vi "csmdoc_load vi description map.vi"(8 "Error in":errorcluster caption="Error in (no error)", 11 "Path":path=path "D:/github/JKI-State-Machine-Plus/.doc/VI Description.md") -> (0 "Error out":errorcluster, 1 "text":string, 2 "variant 2":variant, 3 "variant":variant)   [LabVIEW 2017, in "csmdoc.lvlib"]
uses:
  csmdoc.lvlib
  Communicable State Machine.lvlib
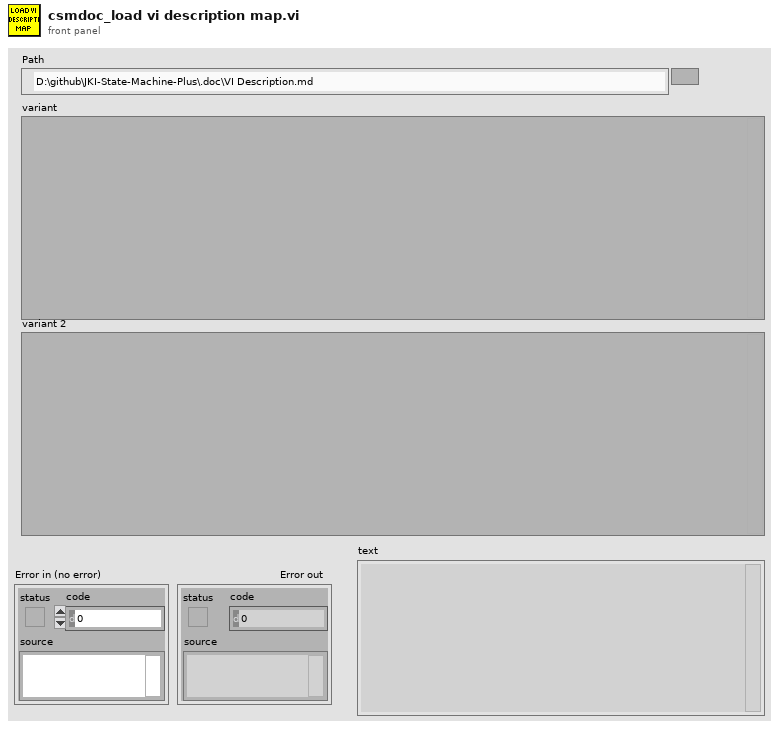
[diagram p1: front panel]
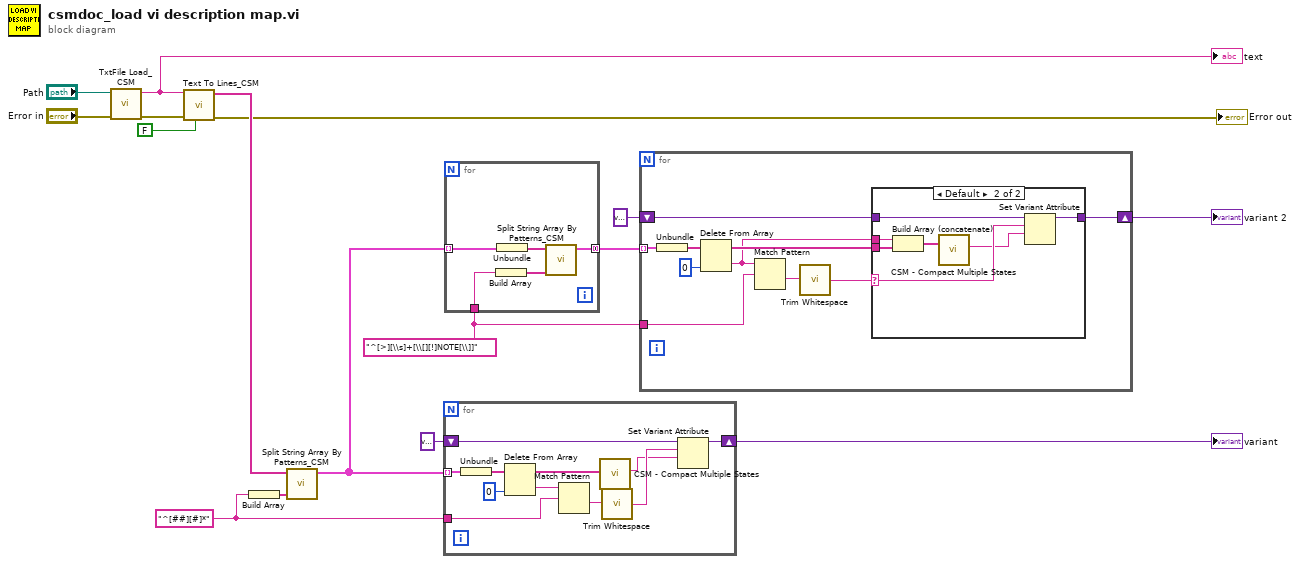
[diagram p0: block diagram]
diagram:
  w2 = "^[>][\\s]+[\\[][!]NOTE[\\]]" ("delimited string")
  w12 = "^[##][#]*" ("delimited string")
  n1 = call "TxtFile Load_CSM.vi"("error in (no error)"="Error in", "Path"="Path") -> ("error out"=w15:errorcluster, "text"=w14:string)  [unwired: 8 in]
  "text" <- w14
  n2 = call "Text To Lines_CSM.vi"("Remove Empty Lines?(T)"=FALSE, "error in (no error)"=w15, "string"=w14) -> ("error out"=→"Error out":errorcluster, "Lines"=w13:string[])  [unwired: 7 in]
  n3 = Build Array(w12) -> (w11:string[])
  n4 = call "Split String Array By Patterns_CSM.vi"("patterns"=w11, "Text Array"=w13) -> ("Array"=w5:cluster{"filtered array":string[]}[])  [unwired: 9 in]
  n5 = for {
    tunnel: w5 -> [w27] mode=indexing
    tunnel: w12 -> [w23]
    shift-right: [w17] -> w9
    shift-left: variant ("variant") -> [w18]
    n6 = Unbundle(w27) -> ("filtered array"=w26:string[])
    n7 = Delete From Array(array=w26, index=0) -> (deleted portion=w24:string, array with subset deleted=w20:string[])  [unwired: 1 in]
    n8 = Match Pattern(string=w24, regular expression=w23) -> (after substring=w22:string)  [unwired: 1 in, 3 out]
    n9 = call "CSM - Compact Multiple States.vi"("Multiple States"=w20) -> ("States"=w19:string)  [unwired: 9 in]
    n10 = call <vilib>:"Trim Whitespace.vi"("string"=w22) -> ("trimmed string"=w21:string)  [unwired: 1 in]
    n11 = Set Variant Attribute(Variant=w18, name=w21, value=w19) -> (Variant out=w17:variant)  [unwired: 1 in, 2 out]
  }
  "variant" <- w9
  n12 = for {
    tunnel: w5 -> [w32] mode=indexing
    tunnel: w2 -> [w30]
    tunnel: [w28] -> w3 mode=concatenating
    n13 = Build Array(w30) -> (w29:string[])
    n14 = Unbundle(w32) -> ("filtered array"=w31:string[])
    n15 = call "Split String Array By Patterns_CSM.vi"("patterns"=w29, "Text Array"=w31) -> ("Array"=w28:cluster{"filtered array":string[]}[])  [unwired: 9 in]
  }
  n16 = for {
    tunnel: w3 -> [w42] mode=indexing
    shift-right: [w36] -> w1
    shift-left: variant ("variant") -> [w37]
    tunnel: w2 -> [w35]
    n17 = Unbundle(w42) -> ("filtered array"=w41:string[])
    n18 = Delete From Array(array=w41, index=0) -> (deleted portion=w33:string, array with subset deleted=w34:string[])  [unwired: 1 in]
    n19 = Match Pattern(string=w33, regular expression=w35) -> (after substring=w39:string)  [unwired: 1 in, 3 out]
    n20 = call <vilib>:"Trim Whitespace.vi"("string"=w39) -> ("trimmed string"=w38:string)  [unwired: 1 in]
    n21 = case shown="Default" w38 {
      selector: w38 -> [_ w50]
      tunnel: w37 -> [w43 w49]
      tunnel: [w43 w48] -> w36
      tunnel: w34 -> [_ w47]
      tunnel: w33 -> [_ w44]
      frame "" {
      }
      frame Default {
        n22 = Build Array (concatenate)(w44, w47) -> (w45:string[])
        n23 = call "CSM - Compact Multiple States.vi"("Multiple States"=w45) -> ("States"=w46:string)  [unwired: 9 in]
        n24 = Set Variant Attribute(Variant=w49, name=w50, value=w46) -> (Variant out=w48:variant)  [unwired: 1 in, 2 out]
      }
    }
  }
  "variant 2" <- w1
